vi "Set Copilot Notifcations.vi"(8 "Error In":errorcluster, 11 "Notification":string) -> (0 "Error Out":errorcluster)   [LabVIEW 2014]
doc: "Dequeues errors for processing\n\nThis VI will block untill an error appears in the Copilot queue."
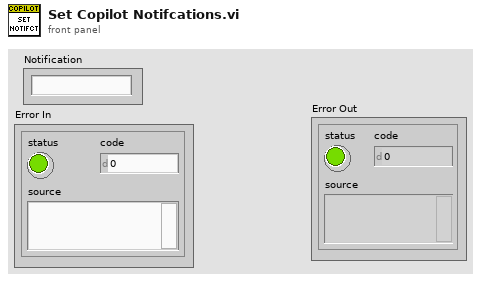
[diagram p1: front panel]
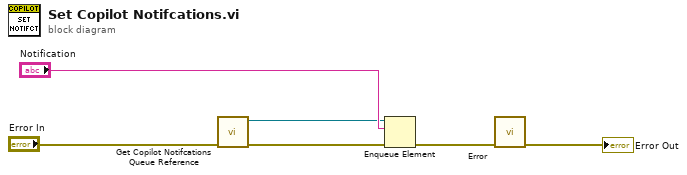
[diagram p0: block diagram]
diagram:
  n1 = call "Get Copilot Notifcations Queue Reference.vi"("Error In"="Error In") -> ("Error Out"=w3:errorcluster, "Co Pilot Notifications Queue Out"=w4:refnum<queue>)  [unwired: 9 in]
  n2 = Enqueue Element(queue=w4, element="Notification", error in (no error)=w3) -> (error out=w6:errorcluster)  [unwired: 1 in, 2 out]
  n3 = call "Error.vi"("Error In"=w6) -> ("Error Out"=→"Error Out":errorcluster)  [unwired: 10 in]
